vi "CtoK.vi"(11 "C":dbl[](array[numeric])) -> (3 "K":dbl[](array[numeric]))   [LabVIEW 2022 SP3]
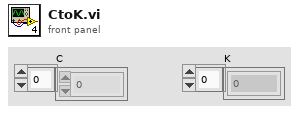
[diagram p1: front panel]
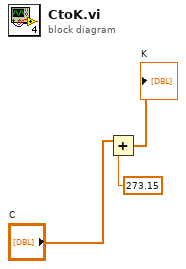
[diagram p0: block diagram]
diagram:
  n1 = Add(x="C", y=273.15) -> (x+y=→"K":dbl[])
